vi "PIDTEMPtest4.vi"() -> ()   [LabVIEW 2015]
uses:
  <vilib>/DAQmx/write.llb/DAQmx Write (Digital 1D Bool NChan 1Samp 1Line).vi
  <vilib>/DAQmx/write.llb/DAQmx Write (Digital Bool 1Line 1Point).vi
  <vilib>/DAQmx/read.llb/DAQmx Read (Analog DBL 1Chan 1Samp).vi
  <vilib>/DAQmx/miscellaneous.llb/DAQmx Fill In Error Info.vi
  <vilib>/addons/control/pid/NI_PID_autopid.lvlib
panel:
  in  "Heater On/Off":bool
  in  "Manual Control":bool
  in  "stop 2":bool
  out "ms to wait":dbl
  out "Control Value":dbl
  in  "setpoint in C":dbl format="%.2f"
  in  "reinitialize? (F)":bool
  in  "autotune? (F)":bool
  out "PID gains out":T1={"proportional gain (Kc)"=1.0, "integral time (Ti, min)"=0.01, "derivative time (Td, min)"=0.0} {"derivative time (Td, min)" format="%.3f"; "integral time (Ti, min)" format="%.3f"; "proportional gain (Kc)" format="%.3f"}
  in  "PID gains":T1={"proportional gain (Kc)"=1.0, "integral time (Ti, min)"=0.01, "derivative time (Td, min)"=0.0} {"derivative time (Td, min)" format="%.3f"; "integral time (Ti, min)" format="%.3f"; "proportional gain (Kc)" format="%.3f"}
  in  "autotuning parameters":T2={"controller type"=1, "relay cycles"=3, "relay amplitude"=1.0, "control specification"=2, "PV noise level"=0.1} {"PV noise level" format="%.2f"; "control specification" items=["normal", "fast", "slow"]; "relay amplitude" format="%.2f"; "controller type" items=["PID", "PI", "P"]}
  in  "stop":bool
  out "Temp":dbl
  out "Temp Chart 2":dbl(graph)
  out "Temp Chart":dbl(graph)
  out "Temp(C)":dbl(slide) scale=-10.0..100.0
  out "Temperature (Celcius)":dbl format="%#.1g"
  out "Voltage Reading(Temp)":dbl format="%#_13g"
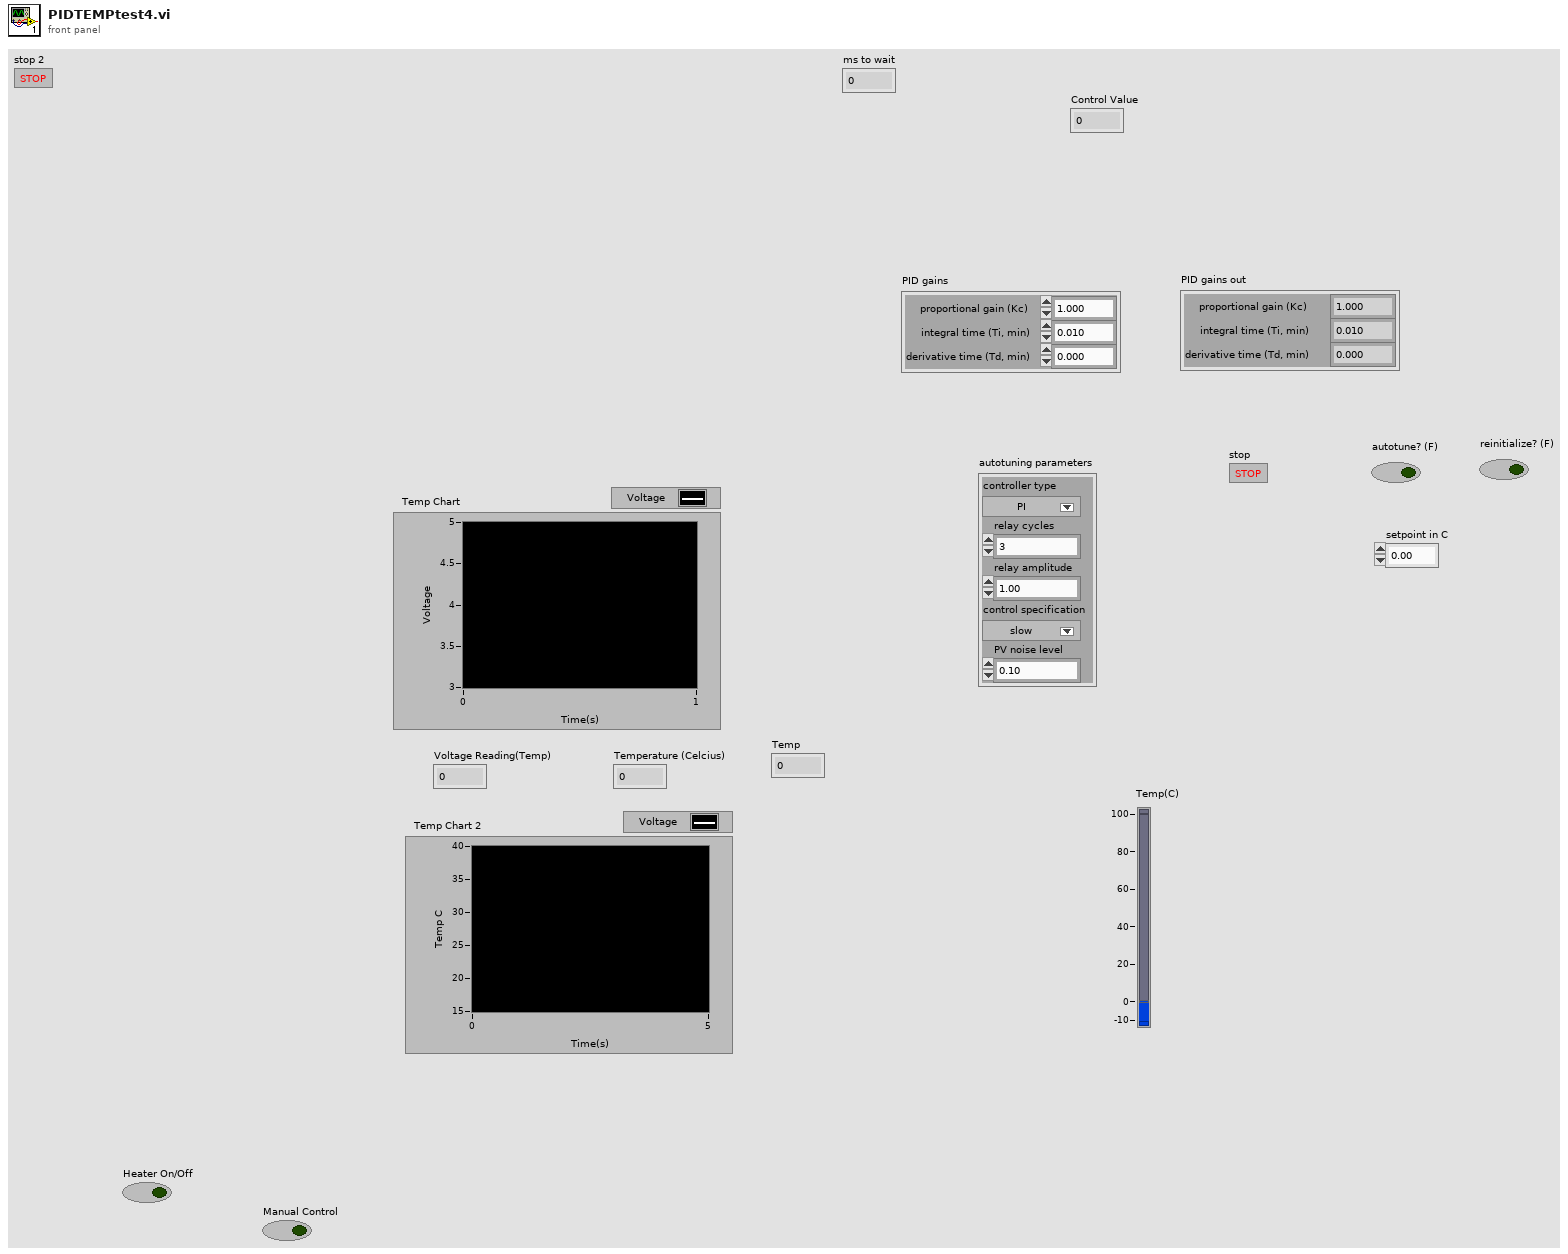
[diagram p1: front panel]
types:
  T1 = cluster{"proportional gain (Kc)":dbl, "integral time (Ti, min)":dbl, "derivative time (Td, min)":dbl}
  T2 = cluster{"controller type":u16, "relay cycles":i32, "relay amplitude":dbl, "control specification":u16, "PV noise level":dbl}
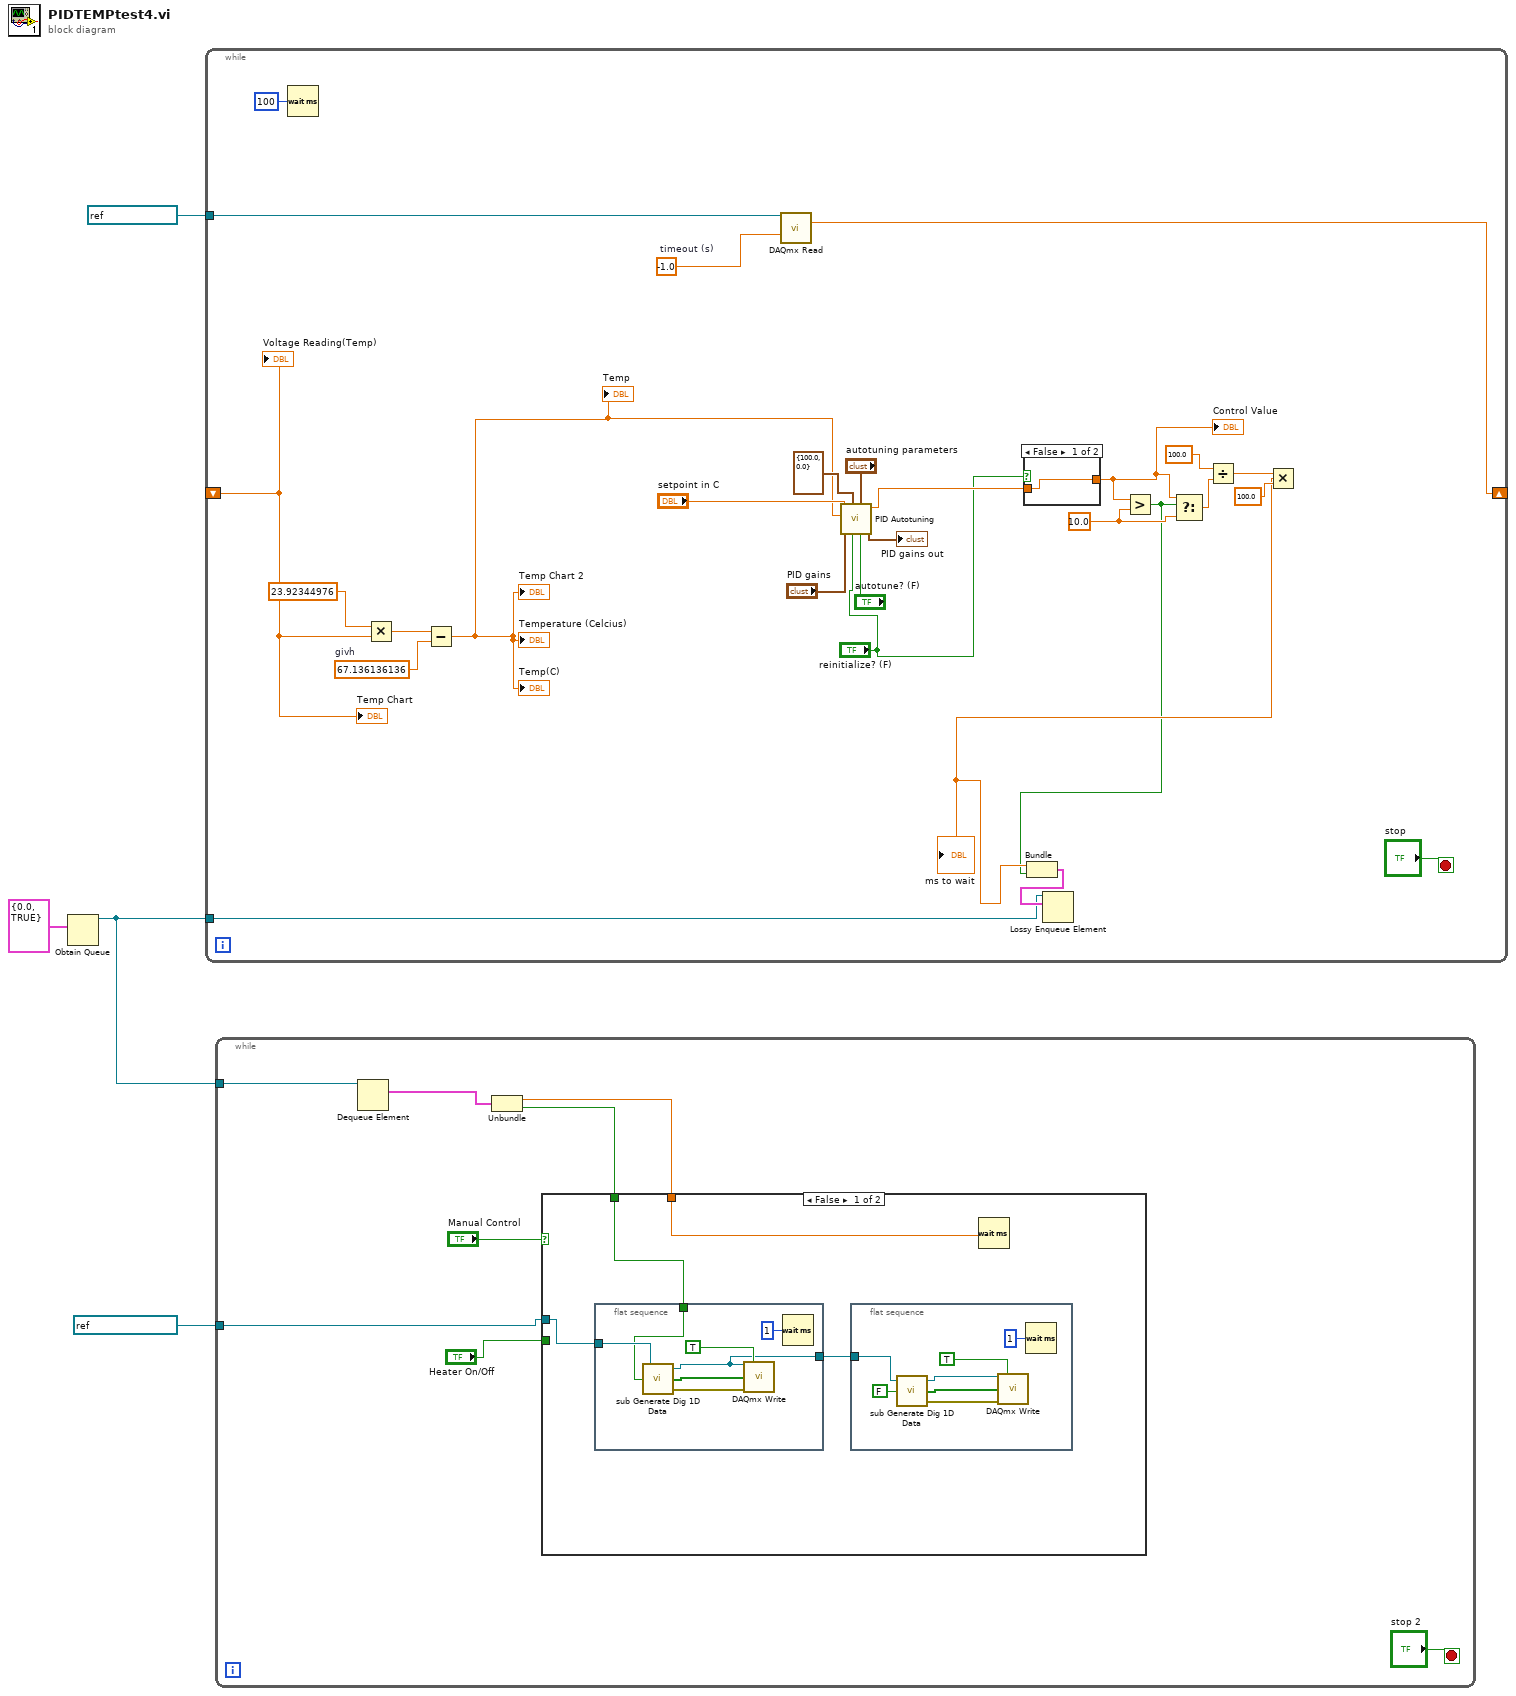
[diagram p0: block diagram]
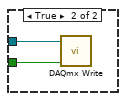
[diagram p2: hidden frame]
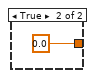
[diagram p3: hidden frame]
diagram:
  n1 = Obtain Queue(element data type=cluster{dbl, bool} {0.0, TRUE}) -> (queue out=w2:refnum<queue>)  [unwired: 4 in, 2 out]
  n2 = while {
    tunnel: refnum<k21> "AnalogInA0" -> [w28]
    shift-right: [w10] -> _
    shift-left: _ -> [w11]
    tunnel: w2 -> [w5]
    stop <- "stop" stop-if-true
    w13 = 10.0 ("f")
    w29 = 67.136136136  # givh
    w32 = -1.0  # timeout (s)
    n3 = Wait (ms)(milliseconds to wait=u32 100) -> ()  [unwired: 1 out]
    n4 = Multiply(x=23.92344976, y=w11) -> (x*y=w30:dbl)
    n5 = Subtract(x=w30, y=w29) -> (x-y=w9:dbl)
    "Temperature (Celcius)" <- w9
    "Temp(C)" <- w9
    "Temp Chart 2" <- w9
    "Temp" <- w9
    n6 = call-poly <vilib>:"DAQmx Read.vi"("task/channels in"=w28, "timeout"=w32) -> ("data"=w10:dbl)  [unwired: 11 in, 2 out]
    n7 = call <vilib>:"PID Autotuning.vi"("autotune? (F)"="autotune? (F)", "autotuning parameters"="autotuning parameters", "reinitialize? (F)"="reinitialize? (F)", "output range"=cluster{"output high":dbl, "output low":dbl} {"output high"=100.0, "output low"=0.0}, "PID gains"="PID gains", "process variable"=w9, "setpoint"="setpoint in C") -> ("PID gains out"=→"PID gains out":T1, "output"=w21:dbl)  [unwired: 1 in, 2 out]
    n8 = case shown="False" "reinitialize? (F)" {
      tunnel: [w33 0.0] -> w14
      tunnel: w21 -> [w33 _]
      frame False {
      }
      frame True {
      }
    }
    "Control Value" <- w14
    n9 = Greater?(x=w14, y=w13) -> (0:w7:bool)
    n10 = Select(t=w14, s=w7, f=w13) -> (s? t:f=w15:dbl)
    n11 = Divide(x=100.0, y=w15) -> (x/y=w17:dbl)
    n12 = Multiply(x=w17, y=100.0) -> (x*y=w8:dbl)
    "ms to wait" <- w8
    n13 = Bundle(w8, w7) -> (w6:cluster{dbl, bool})  [unwired: 1 in]
    n14 = Lossy Enqueue Element(queue=w5, element=w6) -> ()  [unwired: 1 in, 4 out]
    "Voltage Reading(Temp)" <- w11
    "Temp Chart" <- w11
  }
  n15 = while {
    tunnel: w2 -> [w42]
    tunnel: refnum<k21> "YellowdigOUT" -> [w38]
    stop <- "stop 2" stop-if-true
    n16 = Dequeue Element(queue=w42) -> (element=w37:cluster{dbl, bool})  [unwired: 2 in, 3 out]
    n17 = Unbundle(w37) -> (w36:dbl, w35:bool)
    n18 = case shown="False" "Manual Control" {
      tunnel: w38 -> [w45 w62]
      tunnel: "Heater On/Off" -> [_ w61]
      tunnel: w36 -> [w43 _]
      tunnel: w35 -> [w44 _]
      frame False {
        n19 = flat-sequence {
          tunnel: w45 -> [w57]
          tunnel: [w56] -> w46
          tunnel: w44 -> [w55]
          frame #0 {
            n20 = call <vilib>:"sub Generate Dig 1D Data.vi"("initial value"=w55, "task in"=w57) -> ("error out"=w59:errorcluster, "Data"=w60:bool[], "task out"=w56:refnum<k21>)  [unwired: 1 in]
            n21 = call-poly <vilib>:"DAQmx Write.vi"("task/channels in"=w56, "auto start"=TRUE, "data"=w60, "error in"=w59) -> ()  [unwired: 9 in, 3 out]
            n22 = Wait (ms)(milliseconds to wait=u32 1) -> ()  [unwired: 1 out]
          }
        }
        n23 = flat-sequence {
          tunnel: w46 -> [w48]
          frame #0 {
            n24 = call <vilib>:"sub Generate Dig 1D Data.vi"("initial value"=FALSE, "task in"=w48) -> ("error out"=w52:errorcluster, "Data"=w50:bool[], "task out"=w51:refnum<k21>)  [unwired: 1 in]
            n25 = call-poly <vilib>:"DAQmx Write.vi"("task/channels in"=w51, "auto start"=TRUE, "data"=w50, "error in"=w52) -> ()  [unwired: 9 in, 3 out]
            n26 = Wait (ms)(milliseconds to wait=u32 1) -> ()  [unwired: 1 out]
          }
        }
        n27 = Wait (ms)(milliseconds to wait=w43) -> ()  [unwired: 1 out]
      }
      frame True {
        n28 = call-poly <vilib>:"DAQmx Write.vi"("task/channels in"=w62, "data"=w61) -> ()  [unwired: 11 in, 3 out]
      }
    }
  }
